vi "readFromXML.vi"(8 "error in (no error)":errorcluster, 10 "XML in":string, 11 "DifftrackAzEl in":refnum<class "DifftrackAzEl.lvclass">) -> (0 "error out":errorcluster, 3 "DifftrackAzEl out":refnum<class "DifftrackAzEl.lvclass">)   [LabVIEW 2022 SP3, in "TCSDataDefinitions.lvlib" / "TCSCommand.lvlib" / "TargetConfiguration.lvlib" / "Target.lvlib" / "DifftrackAzEl.lvclass"]
uses:
  DifftrackAzEl.lvclass
  <userlib>/Common/UnitsAndXML/FlattenItemWithUnitToXML/FlattenAngularVelocityToXML/AngularVelocityUnit.ctl
  DifftrackAzEl.lvclass/DifftrackAzEl.ctl
  Difftrack.lvclass
  <userlib>/Common/UnitsAndXML/UnitsAndXML.lvlib
  <userlib>/Common/XML/XMLParser/XMLParser.lvclass
panel:
  out "dEl_ArcsPS":dbl[unit]
  out "dAZ_ArcsPS":dbl[unit]
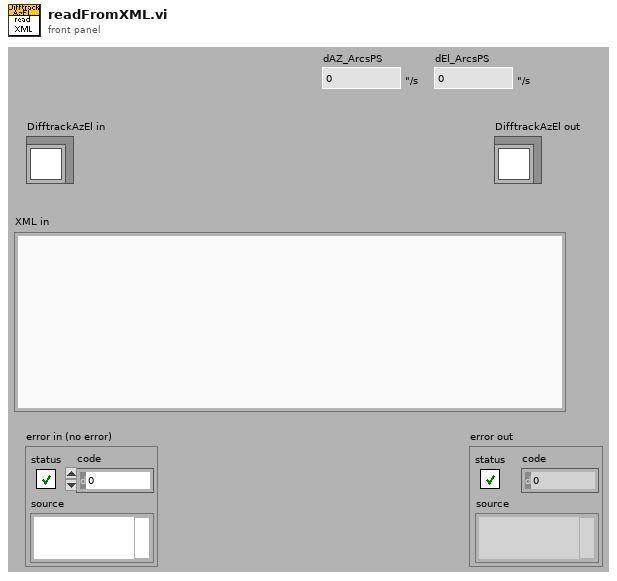
[diagram p1: front panel]
types:
  T1 = typedef "UnitsAndXML.lvlib/AngularVelocityUnit.ctl" = enum16{"\"/a", "deg/s", "\"/s"}
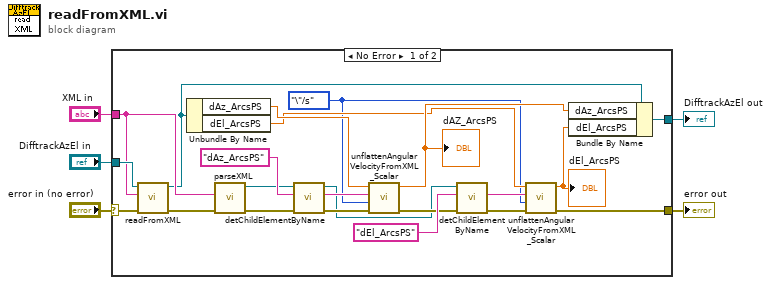
[diagram p0: block diagram]
diagram:
  n1 = case shown="No Error" "error in (no error)" {
    selector: "error in (no error)" -> [w26 w28]
    tunnel: [w10 w28] -> w1
    tunnel: [w20 w29] -> w5
    tunnel: "XML in" -> [w25 _]
    tunnel: "DifftrackAzEl in" -> [w27 w29]
    frame No Error {
      w8 = AngularVelocityUnit."\"/s" ("angularVelocityUnitInXML")
      n2 = call-parent "readFromXML.vi"("error in (no error)"=w26, "XML in"=w25, "Difftrack in"=w27) -> ("error out"=w24:errorcluster, "Difftrack out"=w19:refnum<class "DifftrackAzEl.lvclass">)  [unwired: 7 in]
      n3 = Unbundle By Name(w19) -> ("dAz_ArcsPS"=w18:dbl[unit], "dEl_ArcsPS"=w13:dbl[unit])
      n4 = call <userlib>:"parseXML.vi"("error in (no error)"=w24, "XMLString in"=w25) -> ("error out"=w23:errorcluster, "Element out"=w7:refnum<class "XMLParser.lvclass">)  [unwired: 8 in]
      n5 = call <userlib>:"detChildElementByName.vi"("error in (no error)"=w23, "childName"="dAz_ArcsPS" ("ChildName"), "Element in"=w7) -> ("error out"=w16:errorcluster, "childXML"=w17:string, "Element out"=w6:refnum<class "XMLParser.lvclass">)  [unwired: 5 in, 1 out]
      n6 = call <userlib>:"unflattenAngularVelocityFromXML_Scalar.vi"("error in (no error)"=w16, "angularVelocityUnitInXML"=w8, "xmlString"=w17, "angularVelocityForType"=w18) -> ("error out"=w15:errorcluster, "angularVelocity"=w14:dbl[unit])  [unwired: 6 in]
      "dAZ_ArcsPS" <- w14
      n7 = call <userlib>:"detChildElementByName.vi"("error in (no error)"=w15, "childName"="dEl_ArcsPS" ("ChildName"), "Element in"=w6) -> ("error out"=w11:errorcluster, "childXML"=w9:string)  [unwired: 5 in, 2 out]
      n8 = call <userlib>:"unflattenAngularVelocityFromXML_Scalar.vi"("error in (no error)"=w11, "angularVelocityUnitInXML"=w8, "xmlString"=w9, "angularVelocityForType"=w13) -> ("error out"=w10:errorcluster, "angularVelocity"=w12:dbl[unit])  [unwired: 6 in]
      "dEl_ArcsPS" <- w12
      n9 = Bundle By Name(cluster=w19, "dAz_ArcsPS"=w14, "dEl_ArcsPS"=w12) -> (w20:refnum<class "DifftrackAzEl.lvclass">)
    }
    frame Error {
    }
  }
  "error out" <- w1
  "DifftrackAzEl out" <- w5
